vi "SCD - Read Cookbook.vi"(8 "error in":errorcluster) -> (0 "error out":errorcluster, 1 "Recipe Files":string[](array[string])=["7\t0.02\t999", "5\t0\t-22", "2\t7", "6\t0", "0\t1\t656.20\n0\t1\t656.30\n0\t1\t656.40\n0\t1\t656.50\n0\t1\t656.60\n0\t5\t3", "2\t8", "3\t5", "6\t3", "0\t1\t656.20\n0\t1\t656.30\n0\t1\t656.40\n0\t1\t656.50\n0\t1\t656.60\n0\t5\t3"], 2 "# of Recipes":i16=9, 3 "Cookbook":T1(array[cluster])=[{"Data Type"=enum."SET EXPOSURE", "Arg 1"=0.02, "Arg 2"=999.0, "Arg 3"=path "C:/SCD Cookbooks/scotts_cookbooks/exposure-20ms.rcp", "Comments"=""}, {"Data Type"=enum."MOVE-ABS", "Arg 1"=0.0, "Arg 2"=-22.0, "Arg 3"=path "C:/SCD Cookbooks/scotts_cookbooks/move-absolute-neg22.rcp", "Comments"=""}, {"Data Type"=enum."CAL-FW", "Arg 1"=7.0, "Arg 2"=0.0, "Arg 3"=path "C:/SCD Cookbooks/scotts_cookbooks/cal-dark.rcp", "Comments"=""}, {"Data Type"=enum."DATATYPE", "Arg 1"=0.0, "Arg 2"=0.0, "Arg 3"=path "C:/SCD Cookbooks/scotts_cookbooks/data-type-dark.rcp", "Comments"=""}, {"Data Type"=enum."ACQUIRE DATA", "Arg 1"=5.0, "Arg 2"=3.0, "Arg 3"=path "C:/SCD Cookbooks/scotts_cookbooks/scan-656-5-wavelengths-3-repeats.rcp", "Comments"=""}, {"Data Type"=enum."CAL-FW", "Arg 1"=8.0, "Arg 2"=0.0, "Arg 3"=path "C:/SCD Cookbooks/scotts_cookbooks/cal-open.rcp", "Comments"=""}, {"Data Type"=enum."WAVELENGTH-FW", "Arg 1"=5.0, "Arg 2"=0.0, "Arg 3"=path "C:/SCD Cookbooks/scotts_cookbooks/fw-656.rcp", "Comments"=""}, {"Data Type"=enum."DATATYPE", "Arg 1"=3.0, "Arg 2"=0.0, "Arg 3"=path "C:/SCD Cookbooks/scotts_cookbooks/data-type-obse.rcp", "Comments"=""}, {"Data Type"=enum."ACQUIRE DATA", "Arg 1"=5.0, "Arg 2"=3.0, "Arg 3"=path "C:/SCD Cookbooks/scotts_cookbooks/scan-656-5-wavelengths-3-repeats.rcp", "Comments"=""}], 4 "Cookbook Exposure [ms]":i32=20, 5 "Selected Cookbook":path=path "C:/SCD Cookbooks/scotts_cookbooks/scotts-tester.cbk", 6 "Cookbook Comments":string="* Cookbook Name: scotts-tester.cbk\r\n* Author: S. Sewell\r\n* Date: 2016-Sep-30\r\n* The results of this cookbook should be two large FITS files\r\n*\r\n*\r\n* Set camera exposure to 20ms\r\n*\r\n* Move the camera stage to the best focus position for 656nm\r\n*\r\n* Move the calibration carousel to the dark positon\r\n*\r\n* Set the DataType to 'dark\r\n*\r\n* Acquire a series of images while tuning the Lyot Filter about 656nm\r\n*\r\n* Move the calibration corousel to the open position\r\n*\r\n* Insert the 656nm emission line filter\r\n*\r\n* Set the DataType to 'obse'\r\n*\r\n* Acquire a second series of images again while tuning the Lyot Filter about 656nm\r\n")   [LabVIEW 2014]
uses:
  <vilib>/Utility/file.llb/Read From Spreadsheet File (string).vi
  <vilib>/Utility/file.llb/Read From Spreadsheet File (DBL).vi
panel:
  out "Valid Check":bool[](array[boolean])=[TRUE, TRUE, TRUE, TRUE, TRUE, TRUE, TRUE, TRUE, TRUE]
  out "Recipe Not Found":path
  in  "start path":path=path "C:/SCD Cookbooks/observer"
  in  "Recipe In":T1(array[cluster]) {"Arg 2" format="%.2f"; "Arg 1" format="%.2f"}
  out "List of Recipes":path[](array[path])=[path "C:/SCD Cookbooks/scotts_cookbooks/exposure-20ms.rcp", path "C:/SCD Cookbooks/scotts_cookbooks/move-absolute-neg22.rcp", path "C:/SCD Cookbooks/scotts_cookbooks/cal-dark.rcp", path "C:/SCD Cookbooks/scotts_cookbooks/data-type-dark.rcp", path "C:/SCD Cookbooks/scotts_cookbooks/scan-656-5-wavelengths-3-repeats.rcp", path "C:/SCD Cookbooks/scotts_cookbooks/cal-open.rcp", path "C:/SCD Cookbooks/scotts_cookbooks/fw-656.rcp", path "C:/SCD Cookbooks/scotts_cookbooks/data-type-obse.rcp", path "C:/SCD Cookbooks/scotts_cookbooks/scan-656-5-wavelengths-3-repeats.rcp"]
  # "Arg 1 for a Filter Wheel is the desired position\nArg 1 for Set Exposure is the time in ms\nArg 1 for Acquire Data is the number of images to acquire"
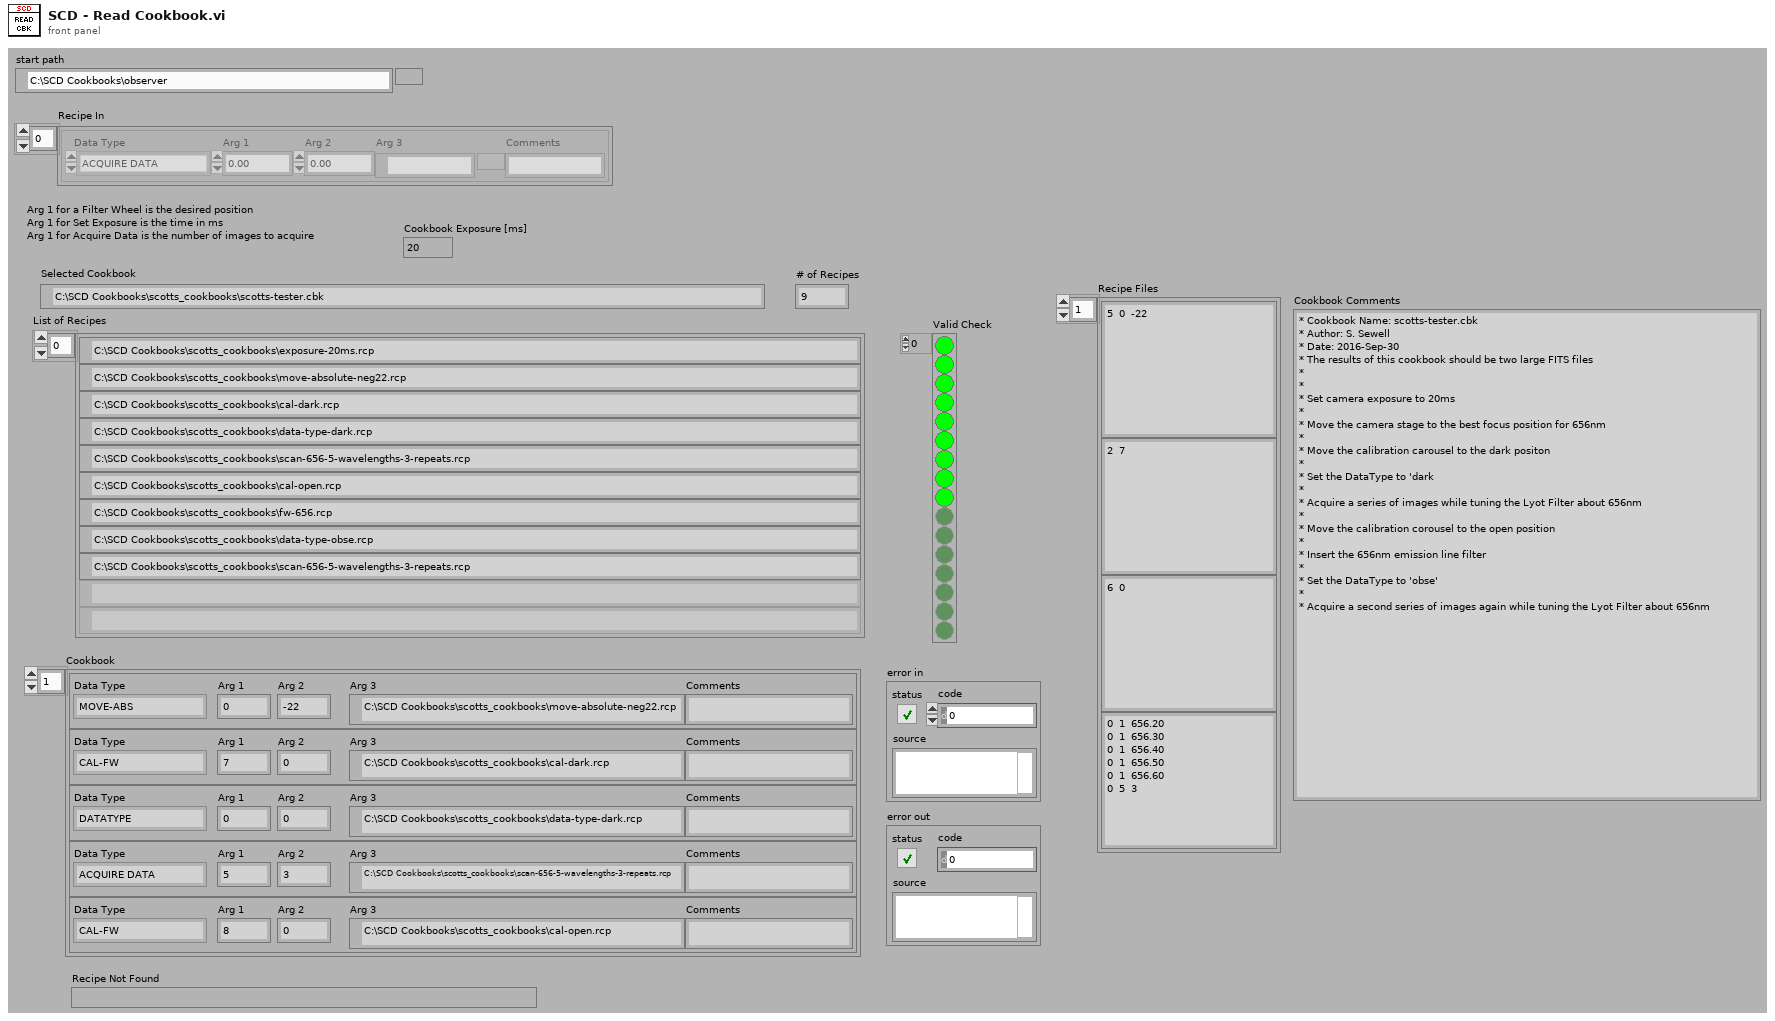
[diagram p1: front panel]
types:
  T1 = cluster{"Data Type":enum32{"ACQUIRE DATA", "SET DIFFUSER", "CAL-FW", "WAVELENGTH-FW", "INSTR. ROTATION", "MOVE-ABS", "DATATYPE", "SET EXPOSURE", "CBK COMMENTS", "MOVE-REL"}, "Arg 1":sgl, "Arg 2":sgl, "Arg 3":path, "Comments":string}[]
  T2 = cluster{"Data Type":enum32{"ACQUIRE DATA", "SET DIFFUSER", "CAL-FW", "WAVELENGTH-FW", "INSTR. ROTATION", "MOVE-ABS", "DATATYPE", "SET EXPOSURE", "CBK COMMENTS", "MOVE-REL"}, "Arg 1":sgl, "Arg 2":sgl, "Arg 3":path, "Comments":string}
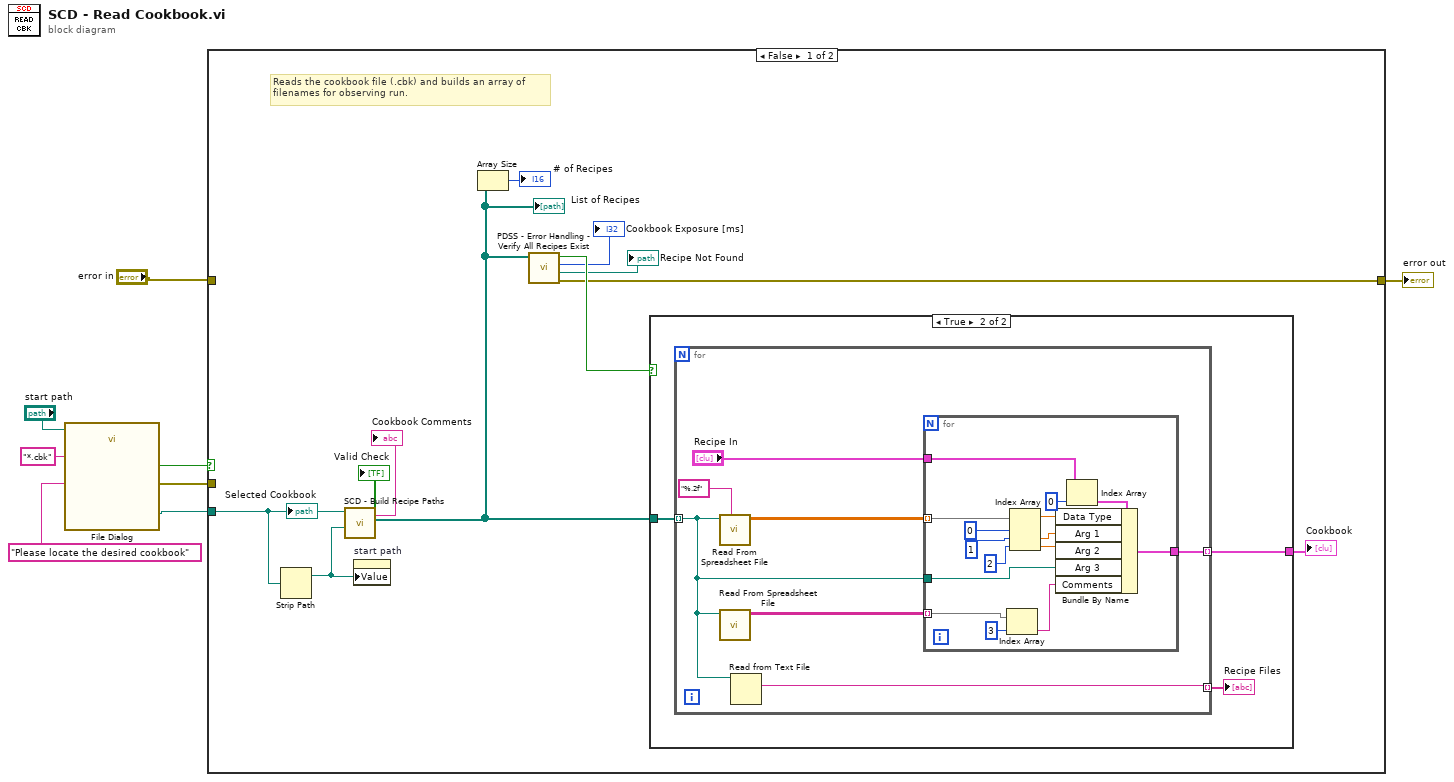
[diagram p0: block diagram]
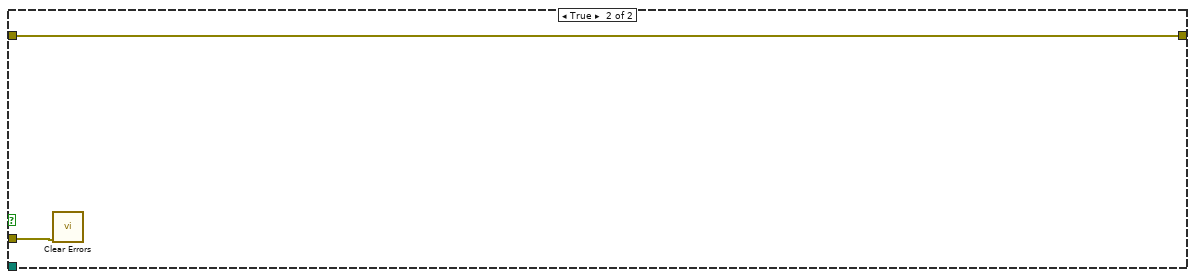
[diagram p3: hidden frame]
diagram:
  n1 = call "File Dialog"("start path"="start path", "prompt"="Please locate the desired cookbook", "pattern (all files)"="*.cbk") -> ("selected path"=w6:path, "cancelled"=w5:bool, "error out"=w1:errorcluster)  [unwired: 4 in, 6 out]
  n2 = case shown="False" w5 {
    tunnel: w6 -> [w10 _]
    tunnel: "error in" -> [_ w46]
    tunnel: [w17 w46] -> w3
    tunnel: w1 -> [_ w45]
    frame False {
      # "Reads the cookbook file (.cbk) and builds an array of\nfilenames for observing run."
      n3 = Strip Path(path=w10) -> (stripped path=w9:path)  [unwired: 1 out]
      n4 = call "SCD - Build Recipe Paths.vi"("Selected path"=w9, "Selected Cookbook"=w10) -> ("Cookbook Recipes"=w11:path[], "Valid Check"=→"Valid Check":bool[], "Cookbook Comments"=→"Cookbook Comments":string)  [unwired: 6 in, 1 out]
      "List of Recipes" <- w11
      n5 = property on="start path" class="Path"("Value"=w9) -> ()  [unwired: 2 in, 2 out]
      n6 = Array Size(array=w11) -> (size(s)=→"# of Recipes":i32)
      n7 = call "PDSS - Error Handling - Verify All Recipes Exist.vi"("List of Recipes"=w11) -> ("error out"=w17:errorcluster, "Recipe Not Found"=→"Recipe Not Found":path, "Max cookbook Exposure [ms]"=→"Cookbook Exposure [ms]":i32, "No errors in cbk"=w18:bool)  [unwired: 7 in]
      n8 = case shown="True" w18 {
        tunnel: [_ w22] -> w16
        tunnel: w11 -> [_ w21]
        frame False {
        }
        frame True {
          n9 = for {
            tunnel: w21 -> [w24] mode=indexing
            tunnel: [w26] -> w22 mode=indexing
            tunnel: [w23] -> w20 mode=indexing
            n10 = call-poly <vilib>:"Read From Spreadsheet File.vi"("format (%.3f)"="%.2f", "file path (dialog if empty)"=w24) -> ("all rows"=w28:dbl[][])  [unwired: 2 in, 7 out]
            n11 = call-poly <vilib>:"Read From Spreadsheet File.vi"("file path (dialog if empty)"=w24) -> ("all rows"=w25:string[][])  [unwired: 6 in, 4 out]
            n12 = Read from Text File(file (use dialog)=w24) -> (text=w23:string)  [unwired: 3 in, 3 out]
            n13 = for {
              tunnel: w28 -> [w44] mode=indexing
              tunnel: "Recipe In" -> [w43]
              tunnel: [w34] -> w26
              tunnel: w24 -> [w33]
              tunnel: w25 -> [w30] mode=indexing
              n14 = Index Array(array=w30, index=3) -> (element=w31:string)
              n15 = Index Array(array=w44, index #1=0 ("index"), index #2=1 ("index"), index #3=2 ("index")) -> (element #1=w39:dbl, element #2=w38:dbl, element #3=w37:dbl)
              n16 = Index Array(array=w43, index=0) -> (element=w35:T2)
              n17 = Bundle By Name(cluster=w35, "Data Type"=w39, "Arg 1"=w38, "Arg 2"=w37, "Arg 3"=w33, "Comments"=w31) -> (w34:T2)
            }
          }
          "Recipe Files" <- w20
        }
      }
      "Cookbook" <- w16
      "Selected Cookbook" <- w10
    }
    frame True {
      n18 = call <vilib>:"Clear Errors.vi"("error in (no error)"=w45) -> ()  [unwired: 5 in, 2 out]
    }
  }
  "error out" <- w3
